vi "Configure Aperture.vi"(5 "Measurement Time (1: Medium)":u16(ring)=1 items=["Short", "Medium", "Long"], 7 "Averaging Factor (1)":i32=1, 8 "error in (no error)":errorcluster, 11 "Agilent 428x in":refnum<class "Agilent 428x.lvclass">) -> (0 "error out":errorcluster, 3 "Agilent 428x out":refnum<class "Agilent 428x.lvclass">)   [LabVIEW 2020, in "Agilent 428x.lvclass"]
uses:
  Agilent 428x.lvclass
  C:/Sandbox/Git_Sandbox/WiSpry Test Framework source code (LV20)/WiSpry Test Framework/Instruments/Instrument.lvclass
  Instrument.lvclass/Instrument.ctl
  Instrument.lvclass
  <instrlib>/Agilent 428X Series/Agilent 428X Series.lvlib
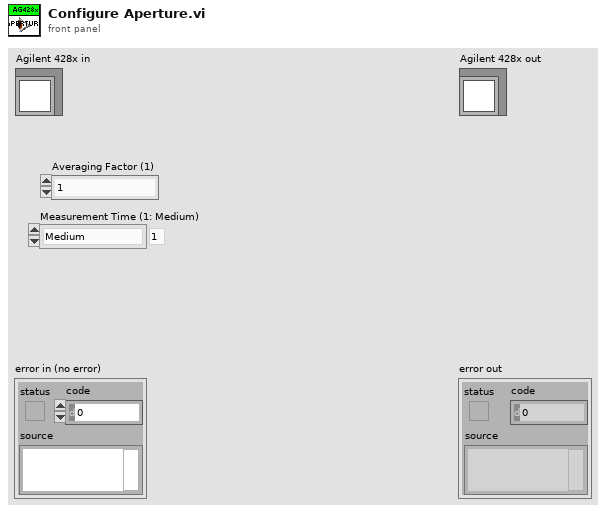
[diagram p1: front panel]
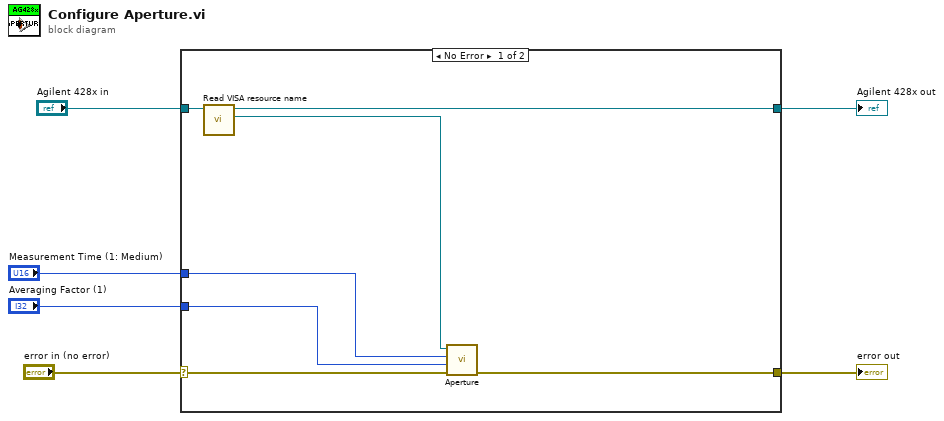
[diagram p0: block diagram]
diagram:
  n1 = case shown="No Error" "error in (no error)" {
    selector: "error in (no error)" -> [w10 w15]
    tunnel: [w9 w15] -> w5
    tunnel: [w12 w14] -> w4
    tunnel: "Agilent 428x in" -> [w13 w14]
    tunnel: "Measurement Time (1: Medium)" -> [w8 _]
    tunnel: "Averaging Factor (1)" -> [w7 _]
    frame No Error {
      n2 = call "Read VISA resource name.vi"("Instrument in"=w13) -> ("VISA resource name"=w11:refnum<visa-resource-name>, "Instrument out"=w12:refnum<class "Agilent 428x.lvclass">)  [unwired: 9 in]
      n3 = call <instrlib>:"Aperture.vi"("error in (no error)"=w10, "Averaging Rate (1)"=w7, "Integ Time (0: Short)"=w8, "VISA resource name"=w11) -> ("error out"=w9:errorcluster)  [unwired: 6 in, 1 out]
    }
    frame Error {
    }
  }
  "error out" <- w5
  "Agilent 428x out" <- w4
